vi "Check position.vi"(8 "error in (no error)":errorcluster, 11 "StageSPIM in":refnum<class "StageSPIM.lvclass">) -> (0 "error out":errorcluster, 3 "StageSPIM out":refnum<class "StageSPIM.lvclass">)   [LabVIEW 2012, in "StageSPIM.lvclass"]
uses:
  StageSPIM.lvclass
  <vilib>/Distrio/Murmex/ProceedMessage/ProceedMessage.lvclass
  <vilib>/Distrio/Murmex/GenericMessage/GenericMessage.lvclass
  StageSPIM.lvclass/StageSPIM.ctl
  <vilib>/Distrio/Murmex/Message/Add or replace parameter.vi
  <vilib>/Distrio/Murmex/Murmex/Murmex.lvclass
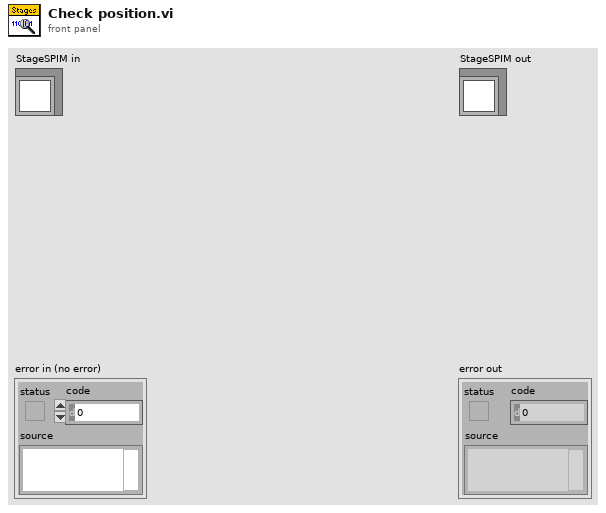
[diagram p1: front panel]
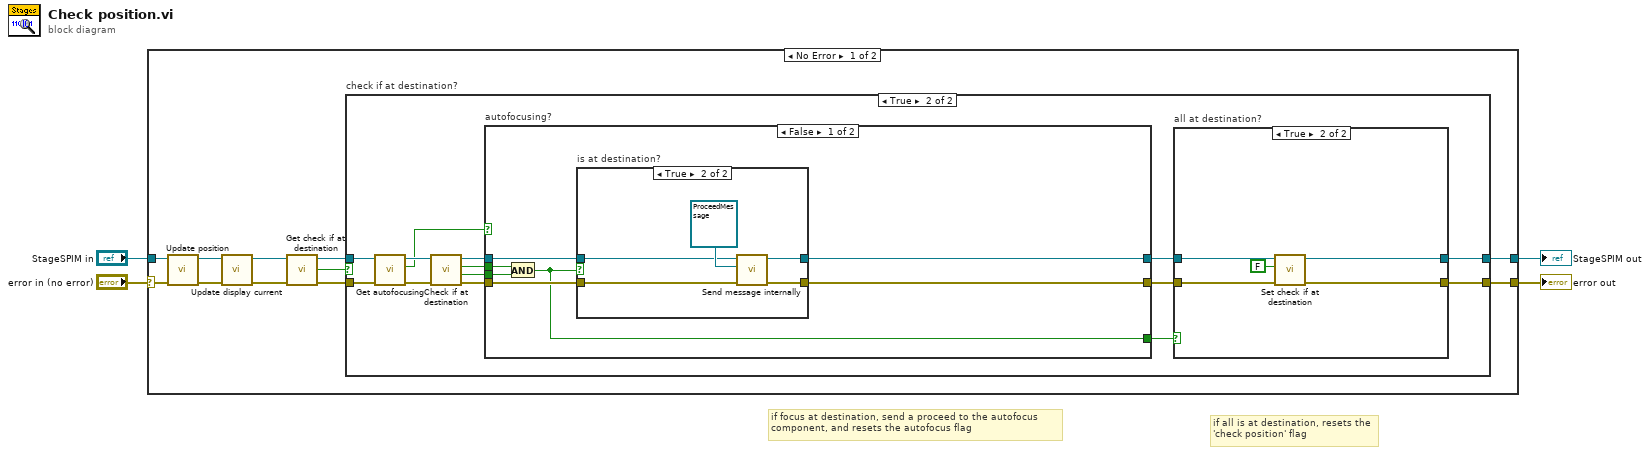
[diagram p0: block diagram]
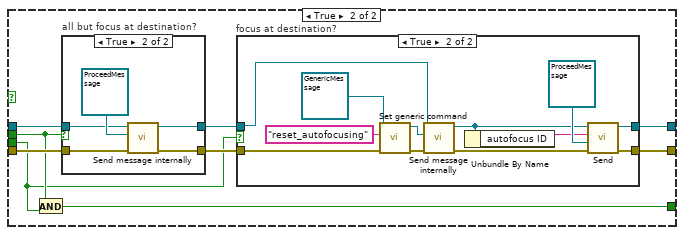
[diagram p5: hidden frame]
diagram:
  # "if all is at destination, resets the\n'check position' flag"
  # "if focus at destination, send a proceed to the autofocus\ncomponent, and resets the autofocus flag"
  n1 = case shown="No Error" "error in (no error)" {
    selector: "error in (no error)" -> [w8 w84]
    tunnel: [w7 w84] -> w3
    tunnel: [w5 w83] -> w1
    tunnel: "StageSPIM in" -> [w6 w83]
    frame No Error {
      n2 = call-dynamic "Update position.vi"("error in (no error)"=w8, "StageSPIM in"=w6) -> ("error out"=w12:errorcluster, "StageSPIM out"=w10:refnum<class "StageSPIM.lvclass">)  [unwired: 8 in]
      n3 = call-dynamic "Update display current.vi"("error in (no error)"=w12, "StageSPIM in"=w10) -> ("error out"=w11:errorcluster, "StageSPIM out"=w9:refnum<class "StageSPIM.lvclass">)  [unwired: 8 in]
      n4 = call-dynamic "Get check if at destination.vi"("error in (no error)"=w11, "StageSPIM in"=w9) -> ("error out"=w14:errorcluster, "check if at destination"=w15:bool, "StageSPIM out"=w13:refnum<class "StageSPIM.lvclass">)  [unwired: 7 in]
      n5 = case "check if at destination?" shown="True" w15 {
        tunnel: w14 -> [w17 w28]
        tunnel: w13 -> [w16 w26]
        tunnel: [w16 w20] -> w5
        tunnel: [w17 w19] -> w7
        frame False {
        }
        frame True {
          n6 = call-dynamic "Get autofocusing.vi"("error in (no error)"=w28, "StageSPIM in"=w26) -> ("error out"=w27:errorcluster, "autofocusing?"=w24:bool, "StageSPIM out"=w25:refnum<class "StageSPIM.lvclass">)  [unwired: 7 in]
          n7 = call-dynamic "Check if at destination.vi"("error in (no error)"=w27, "StageSPIM in"=w25) -> ("error out"=w30:errorcluster, "focus at destination?"=w23:bool, "at destination? (all but focus)"=w31:bool, "StageSPIM out"=w29:refnum<class "StageSPIM.lvclass">)  [unwired: 6 in]
          n8 = case "autofocusing?" shown="False" w24 {
            tunnel: w31 -> [w41 w57]
            tunnel: w30 -> [w45 w61]
            tunnel: w29 -> [w44 w60]
            tunnel: [w43 w55] -> w22
            tunnel: [w42 w54] -> w21
            tunnel: w23 -> [w40 w56]
            tunnel: [w39 w53] -> w18
            frame False {
              n9 = And(x=w41, y=w40) -> (x .and. y?=w39:bool)
              n10 = case "is at destination?" shown="True" w39 {
                tunnel: w45 -> [w47 w48]
                tunnel: w44 -> [w46 w49]
                tunnel: [w47 w51] -> w42
                tunnel: [w46 w50] -> w43
                frame False {
                }
                frame True {
                  n11 = call <vilib>:"Send message internally.vi"("error in (no error)"=w48, "Message"=refnum<class "ProceedMessage.lvclass"> refnum ("Distrio Murmex 1.1:ProceedMessage"), "Murmex in"=w49) -> ("error out"=w51:errorcluster, "Murmex out"=w50:refnum<class "StageSPIM.lvclass">)  [unwired: 7 in]
                }
              }
            }
            frame True {
              n12 = And(x=w57, y=w56) -> (x .and. y?=w53:bool)
              n13 = case "all but focus at destination?" shown="True" w57 {
                tunnel: w61 -> [w77 w78]
                tunnel: w60 -> [w76 w79]
                tunnel: [w77 w81] -> w58
                tunnel: [w76 w80] -> w59
                frame False {
                }
                frame True {
                  n14 = call <vilib>:"Send message internally.vi"("error in (no error)"=w78, "Message"=refnum<class "ProceedMessage.lvclass"> refnum ("Distrio Murmex 1.1:ProceedMessage"), "Murmex in"=w79) -> ("error out"=w81:errorcluster, "Murmex out"=w80:refnum<class "StageSPIM.lvclass">)  [unwired: 7 in]
                }
              }
              n15 = case "focus at destination?" shown="True" w56 {
                tunnel: w58 -> [w63 w69]
                tunnel: w59 -> [w62 w66]
                tunnel: [w63 w72] -> w54
                tunnel: [w62 w73] -> w55
                frame False {
                }
                frame True {
                  n16 = call <vilib>:"Set generic command.vi"("error in (no error)"=w69, "generic command"="reset_autofocusing", "GenericMessage in"=refnum<class "GenericMessage.lvclass"> refnum ("Message in")) -> ("error out"=w70:errorcluster, "GenericMessage out"=w65:refnum<class "GenericMessage.lvclass">)  [unwired: 7 in]
                  n17 = call <vilib>:"Send message internally.vi"("error in (no error)"=w70, "Message"=w65, "Murmex in"=w66) -> ("error out"=w68:errorcluster, "Murmex out"=w67:refnum<class "StageSPIM.lvclass">)  [unwired: 7 in]
                  n18 = Unbundle By Name(w67) -> ("autofocus ID"=w74:string)
                  n19 = call <vilib>:"Send.vi"("error in (no error)"=w68, "Message"=refnum<class "ProceedMessage.lvclass"> refnum ("Distrio Murmex 1.1:ProceedMessage"), "recipient"=w74, "Murmex in"=w67) -> ("error out"=w72:errorcluster, "Murmex out"=w73:refnum<class "StageSPIM.lvclass">)  [unwired: 6 in]
                }
              }
            }
          }
          n20 = case "all at destination?" shown="True" w18 {
            tunnel: w22 -> [w33 w36]
            tunnel: w21 -> [w32 w38]
            tunnel: [w33 w35] -> w20
            tunnel: [w32 w37] -> w19
            frame False {
            }
            frame True {
              n21 = call-dynamic "Set check if at destination.vi"("error in (no error)"=w38, "check if at destination"=FALSE, "StageSPIM in"=w36) -> ("error out"=w37:errorcluster, "StageSPIM out"=w35:refnum<class "StageSPIM.lvclass">)  [unwired: 7 in]
            }
          }
        }
      }
    }
    frame Error {
    }
  }
  "error out" <- w3
  "StageSPIM out" <- w1
